vi "Get OUT16 Measure Data Size.vi"() -> (0 "OUT16 Measure Data Size":u32)   [LabVIEW 8.6, in "Keyence LJ-V7000.lvlib"]
uses:
  Keyence LJ-V7000.lvlib
  Public/constant/Judge Result.ctl
  Public/constant/Measure Data Info.ctl
  Public/Clusters/Measure Data.ctl
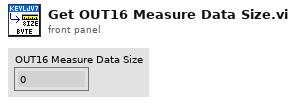
[diagram p1: front panel]
types:
  T1 = typedef "Keyence LJ-V7000.lvlib/Measure Data.ctl" = cluster{"Data Info":T2, "Judge Result":T3, "reserve":u8, "reserve":u8, "Value":sgl}
  T2 = typedef "Keyence LJ-V7000.lvlib/Measure Data Info.ctl" = u8
  T3 = typedef "Keyence LJ-V7000.lvlib/Judge Result.ctl" = u8
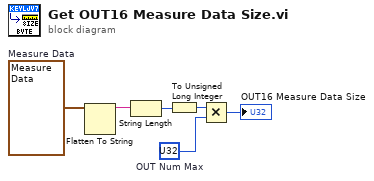
[diagram p0: block diagram]
diagram:
  w3 = u32 ?  # OUT Num Max
  w1 = T1 ?  # Measure Data
  n1 = Flatten To String(anything=w1) -> (data string=w2:string)  [unwired: 3 in, 2 out]
  n2 = String Length(string=w2) -> (length=w6:i32)
  n3 = To Unsigned Long Integer(number=w6) -> (unsigned 32bit integer=w5:u32)
  n4 = Multiply(x=w5, y=w3) -> (x*y=→"OUT16 Measure Data Size":u32)
